vi "Open_CCS_Handle.vi"(0 "Labview-T/Teststand-F":bool=TRUE, 1 "Input_Files":T1={"CCS Base Folder"=path "C:/ti/ccs1120/ccs/ccs_base", "CCXML File (target configuration)"=path "C:/Users/wcslab/ti/CCSTargetConfigurations/CC23405R.ccxml", "Projects Folder"=path "C:/Users/wcslab/workspace_v2/adc_wakeup_time/Debug/adc_wakeup_time.out"}, 5 "error in (no error)":errorcluster) -> (14 "Boolean":bool=TRUE, 19 "error out":errorcluster)   [LabVIEW 2019]
uses:
  <userlib>/_TI-LA/Reusable/CCS/APIs/CCS.lvlib
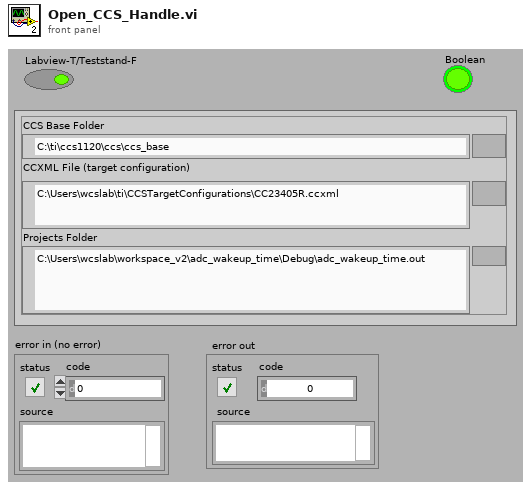
[diagram p1: front panel]
types:
  T1 = cluster{"CCS Base Folder":path, "CCXML File (target configuration)":path, "Projects Folder":path}
  T2 = cluster{"Core Number":u16, "Port Number":u16, "Run Minimized? (F)":bool, "Quiet Frame? (F)":bool, "Host Name":string}
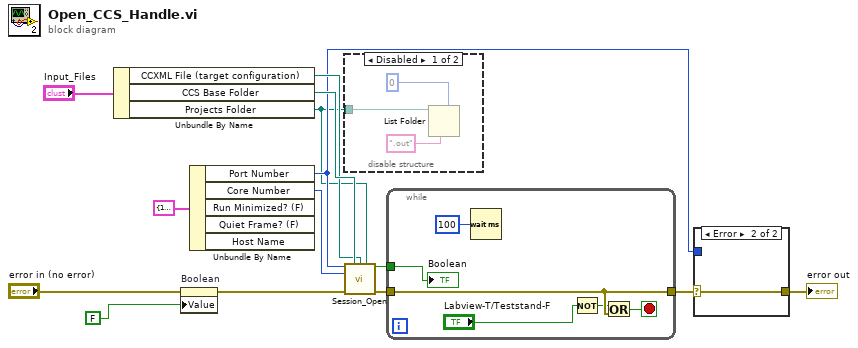
[diagram p0: block diagram]
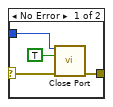
[diagram p3: hidden frame]
diagram:
  n1 = Unbundle By Name("Input_Files") -> ("CCXML File (target configuration)"=w6:path, "CCS Base Folder"=w7:path, "Projects Folder"=w1:path)
  n2 = property on="Boolean" class="Bool (strict)"(error in="error in (no error)", "Value"=FALSE ("Boolean")) -> (error out=w8:errorcluster)  [unwired: 1 in, 1 out]
  n3 = Unbundle By Name(T2 {"Core Number"=1, "Port Number"=1444, "Run Minimized? (F)"=TRUE, "Quiet Frame? (F)"=TRUE, "Host Name"="localhost"}) -> ("Port Number"=w2:u16, "Core Number"=w5:u16)  [unwired: 3 out]
  n4 = disable-structure shown="Disabled" {
    disable-tunnel: w1 -> [w17 _]
    frame Disabled {
      n5 = List Folder(datalog type=0, path=w17, pattern=".out") -> ()  [unwired: 1 in, 4 out]
    }
    frame Enabled {
    }
  }
  n6 = call "Session_Open.vi"("Port Number"=w2, "CCS Base Folder 2"=w7, "CCXML File (target configuration)"=w6, "program file"=w1, "Core Number"=w5, "error in (no error)"=w8) -> ("Programed"=w4:bool, "error out"=w3:errorcluster)  [unwired: 8 in]
  n7 = while {
    tunnel: w3 -> [w21]
    tunnel: [w21] -> w12
    tunnel: w4 -> [w18]
    stop <- w22 stop-if-true
    n8 = Wait (ms)(milliseconds to wait=u32 100) -> ()  [unwired: 1 out]
    n9 = Not(x="Labview-T/Teststand-F") -> (.not. x?=w19:bool)
    n10 = Or(x=w19, y=w21) -> (x .or. y?=w22:bool)
    "Boolean" <- w18
  }
  n11 = case shown="Error" w12 {
    selector: w12 -> [w25 w28]
    tunnel: w2 -> [w27 _]
    tunnel: [w24 w28] -> w11
    frame No Error {
      n12 = call <userlib>:"Close Port.vi"("Port Number"=w27, "Kill Sessions? (F)"=TRUE, "error in"=w25) -> ("error out"=w24:errorcluster)  [unwired: 10 in, 2 out]
    }
    frame Error {
    }
  }
  "error out" <- w11
